vi "Stop Process VI.vi"(8 "error in (no error)":errorcluster, 9 "Blocking (T)":bool=TRUE, 10 "Process Name":string, 11 "Data in":T1={"Main VI Queue"=refnum, "Process Queue References"=[], "Message Queue"=refnum, "Visible Hardware VI"="", "Current Message"={"Source"="", "Destination"="", "Time Stamp"=timestamp(0 s since 1904-01-01), "Command"="", "Data"=variant(string "")}, "Message History"=[], "Hardware"={"Process Cache"=refnum, "Plugins"=[{"Plugin Name"="", "Controller Type"=enum."Invalid", "Control Panel Path"=path "", "Plugin Type"=enum."Optimizer"}, {"Plugin Name"="", "Controller Type"=enum."Invalid", "Control Panel Path"=path "", "Plugin Type"=enum."Optimizer"}, {"Plugin Name"="", "Controller Type"=enum."Invalid", "Control Panel Path"=path "", "Plugin Type"=enum."Optimizer"}, {"Plugin Name"="", "Controller Type"=enum."Invalid", "Control Panel Path"=path "", "Plugin Type"=enum."Optimizer"}]}, "Optimizers"={"Process Cache"=refnum, "Plugins"=[{"Plugin Name"="Deep Reaction Optimizer", "Controller Type"=enum."Invalid", "Control Panel Path"=path "", "Plugin Type"=enum."Optimizer"}, {"Plugin Name"="..\\Optimizers\\Deep Reaction Optimizer\\Control Panel\\Main.vi", "Controller Type"=enum."Invalid", "Control Panel Path"=path "", "Plugin Type"=enum."Optimizer"}, {"Plugin Name"="..\\Optimizers\\Deep Reaction Optimizer\\Source - zmq\\start_inference.bat", "Controller Type"=enum."Invalid", "Control Panel Path"=path "", "Plugin Type"=enum."Optimizer"}], "First parameters?"=FALSE, "New Parameters"={"Time Stamp"=timestamp(0 s since 1904-01-01), "Names"=[], "Values"=[]}}, "Parameter to Hardware Map"=refnum, "Analyzers"={"Process Cache"=refnum, "Plugins"=[{"Plugin Name"="ChromTech Pump Controller", "Controller Type"=enum."Invalid", "Control Panel Path"=path "", "Plugin Type"=enum."Optimizer"}, {"Plugin Name"="Pump Controller", "Controller Type"=enum."Invalid", "Control Panel Path"=path "", "Plugin Type"=enum."Optimizer"}, {"Plugin Name"="..\\Instrumentation\\ChromTech MX-Class\\Control Panel\\Main.vi", "Controller Type"=enum."Invalid", "Control Panel Path"=path "", "Plugin Type"=enum."Optimizer"}, {"Plugin Name"="", "Controller Type"=enum."Invalid", "Control Panel Path"=path "", "Plugin Type"=enum."Optimizer"}]}, "Log Directory"=path "", "Auto Pass Parameters"=FALSE, "Experiment"={"Name"="", "File Path"=path "", "File Extension"="", "File Cluster"={"Hardware List"=[], "Optimizer List"=[], "Analyzer List"=[], "Parameter to Hardware Map"=[]}}}) -> (0 "error out":errorcluster, 3 "Data out":T1={"Main VI Queue"=refnum, "Process Queue References"=[], "Message Queue"=refnum, "Visible Hardware VI"="", "Current Message"={"Source"="", "Destination"="", "Time Stamp"=timestamp(0 s since 1904-01-01), "Command"="", "Data"=variant(string "")}, "Message History"=[], "Hardware"={"Process Cache"=refnum, "Plugins"=[{"Plugin Name"="", "Controller Type"=enum."Invalid", "Control Panel Path"=path "", "Plugin Type"=enum."Optimizer"}, {"Plugin Name"="", "Controller Type"=enum."Invalid", "Control Panel Path"=path "", "Plugin Type"=enum."Optimizer"}, {"Plugin Name"="", "Controller Type"=enum."Invalid", "Control Panel Path"=path "", "Plugin Type"=enum."Optimizer"}, {"Plugin Name"="", "Controller Type"=enum."Invalid", "Control Panel Path"=path "", "Plugin Type"=enum."Optimizer"}]}, "Optimizers"={"Process Cache"=refnum, "Plugins"=[{"Plugin Name"="Deep Reaction Optimizer", "Controller Type"=enum."Invalid", "Control Panel Path"=path "", "Plugin Type"=enum."Optimizer"}, {"Plugin Name"="..\\Optimizers\\Deep Reaction Optimizer\\Control Panel\\Main.vi", "Controller Type"=enum."Invalid", "Control Panel Path"=path "", "Plugin Type"=enum."Optimizer"}, {"Plugin Name"="..\\Optimizers\\Deep Reaction Optimizer\\Source - zmq\\start_inference.bat", "Controller Type"=enum."Invalid", "Control Panel Path"=path "", "Plugin Type"=enum."Optimizer"}], "First parameters?"=FALSE, "New Parameters"={"Time Stamp"=timestamp(0 s since 1904-01-01), "Names"=[], "Values"=[]}}, "Parameter to Hardware Map"=refnum, "Analyzers"={"Process Cache"=refnum, "Plugins"=[{"Plugin Name"="ChromTech Pump Controller", "Controller Type"=enum."Invalid", "Control Panel Path"=path "", "Plugin Type"=enum."Optimizer"}, {"Plugin Name"="Pump Controller", "Controller Type"=enum."Invalid", "Control Panel Path"=path "", "Plugin Type"=enum."Optimizer"}, {"Plugin Name"="..\\Instrumentation\\ChromTech MX-Class\\Control Panel\\Main.vi", "Controller Type"=enum."Invalid", "Control Panel Path"=path "", "Plugin Type"=enum."Optimizer"}, {"Plugin Name"="", "Controller Type"=enum."Invalid", "Control Panel Path"=path "", "Plugin Type"=enum."Optimizer"}]}, "Log Directory"=path "", "Auto Pass Parameters"=FALSE, "Experiment"={"Name"="", "File Path"=path "", "File Extension"="", "File Cluster"={"Hardware List"=[], "Optimizer List"=[], "Analyzer List"=[], "Parameter to Hardware Map"=[]}}})   [LabVIEW 2020]
doc: "Stops the named process, shutting down the subpanel indicator and control panel, removing the entry from the message history cache, and deleting it form the object array. This VI triggers status update events."
uses:
  Plugin Servers/Controller Array/Controller Array.lvclass
  Type Definitions/Data.ctl
  Plugin Servers/Parameter to Hardware Map/Parameter to Hardware Map.lvclass
  <userlib>/Dynamic Reentrant/Type Defs/Message.ctl
  Plugin Manager/Plugin Details.ctl
  Plugin Servers/Controller/Controller Type.ctl
  Plugin Manager/Plugin Types.ctl
  Experiment/Experiment File/Experiment File Cluster.ctl
  Plugin Servers/Controller/Minimal Controller Cluster.ctl
  Plugin Servers/Parameter to Hardware Map/Minimal Map.ctl
  Plugin Servers/Parameter to Hardware Map/Minimal Pair Cluster.ctl
  Plugin Servers/Controller/Generic Plugin.lvclass
  <userlib>/Dynamic Reentrant/Dynamic Reentrant.lvlib
  Experiment/Experiment File/Experiment File.lvlib
  Plugin Manager/Plugin Manager.lvlib
panel:
  # "Note: Rxn Rover data control and indicator have been hidden!"
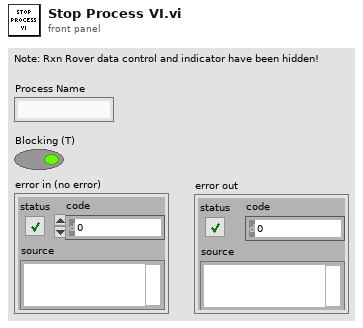
[diagram p1: front panel]
types:
  T1 = typedef "Data.ctl" = cluster{"Main VI Queue":refnum<queue>, "Process Queue References":refnum<queue>[], "Message Queue":refnum<queue>, "Visible Hardware VI":string, "Current Message":T2, "Message History":string[][], "Hardware":cluster{"Process Cache":refnum<class "Controller Array.lvclass">, "Plugins":T3[]}, "Optimizers":cluster{"Process Cache":refnum<class "Controller Array.lvclass">, "Plugins":T3[], "First parameters?":bool, "New Parameters":cluster{"Time Stamp":timestamp, "Names":string[], "Values":dbl[]}}, "Parameter to Hardware Map":refnum<class "Parameter to Hardware Map.lvclass">, "Analyzers":cluster{"Process Cache":refnum<class "Controller Array.lvclass">, "Plugins":T3[]}, "Log Directory":path, "Auto Pass Parameters":bool, "Experiment":cluster{"Name":string, "File Path":path, "File Extension":string, "File Cluster":T6}}
  T2 = typedef "Dynamic Reentrant.lvlib/Message.ctl" = cluster{"Source":string, "Destination":string, "Time Stamp":timestamp, "Command":string, "Data":variant}
  T3 = typedef "Plugin Manager.lvlib/Plugin Details.ctl" = cluster{"Plugin Name":string, "Controller Type":T4, "Control Panel Path":path, "Plugin Type":T5}
  T4 = typedef "Generic Plugin.lvclass/Controller Type.ctl" = enum16{"Invalid", "Temperature Controller", "Pump Controller", "Generic Optimizer", "LC Parser"}
  T5 = typedef "Plugin Manager.lvlib/Plugin Types.ctl" = enum16{"Invalid", "Optimizer", "Analyzer", "Hardware"}
  T6 = typedef "Experiment File.lvlib/Experiment File Cluster.ctl" = cluster{"Hardware List":T7[], "Optimizer List":T7[], "Analyzer List":T7[], "Parameter to Hardware Map":T8}
  T7 = typedef "Generic Plugin.lvclass/Minimal Controller Cluster.ctl" = cluster{"Name":string, "Controller Type":string, "Control Panel Path":string, "Resource":string}
  T8 = typedef "Parameter to Hardware Map.lvclass/Minimal Map.ctl" = T9[]
  T9 = typedef "Parameter to Hardware Map.lvclass/Minimal Pair Cluster.ctl" = cluster{"key":string, "values":T7[]}
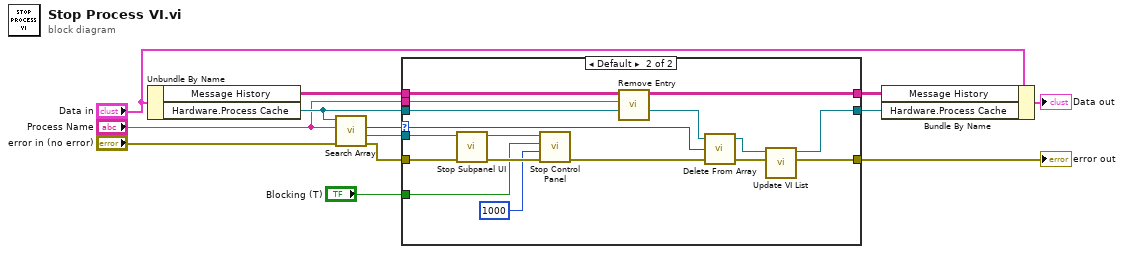
[diagram p0: block diagram]
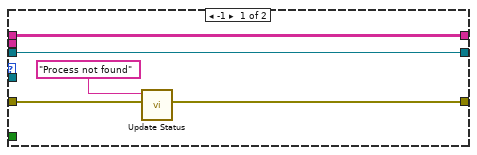
[diagram p2: hidden frame]
diagram:
  n1 = Unbundle By Name("Data in") -> ("Message History"=w7:string[][], "Hardware.Process Cache"=w8:refnum<class "Controller Array.lvclass">)
  n2 = call "Search Array.vi"("error in (no error)"="error in (no error)", "Search Value"="Process Name", "Controller Array in"=w8) -> ("error out"=w10:errorcluster, "Controller found"=w11:refnum<class "Generic Plugin.lvclass">, "Index of found"=w9:i32)  [unwired: 1 in, 1 out]
  n3 = case shown="Default" w9 {
    selector: w9 -> [_ w30]
    tunnel: [w17 w20] -> w13
    tunnel: w11 -> [_ w33]
    tunnel: w10 -> [w18 w31]
    tunnel: w8 -> [w15 w29]
    tunnel: [w15 w26] -> w3
    tunnel: w7 -> [w14 w25]
    tunnel: "Process Name" -> [_ w24]
    tunnel: [w14 w23] -> w4
    tunnel: "Blocking (T)" -> [_ w21]
    frame -1 {
      n4 = call "Update Status.vi"("error in (no error)"=w18, "Status Bar Text"="Process not found") -> ("error out"=w17:errorcluster)  [unwired: 9 in]
    }
    frame Default {
      n5 = call "Stop Subpanel UI.vi"("error in (no error)"=w31, "Controller in"=w33) -> ("error out"=w34:errorcluster, "Controller out"=w32:refnum<class "Generic Plugin.lvclass">)  [unwired: 8 in]
      n6 = call "Stop Control Panel.vi"("error in (no error)"=w34, "timeout in ms (-1)"=1000, "Blocking (T)"=w21, "controller in"=w32) -> ("error out"=w22:errorcluster)  [unwired: 6 in, 1 out]
      n7 = call "Remove Entry.vi"("Source"=w24, "Message History in"=w25) -> ("Message History out"=w23:string[][])  [unwired: 9 in]
      n8 = call "Delete From Array.vi"("error in (no error)"=w22, "index (last elem)"=w30, "Controller Array in"=w29) -> ("error out"=w27:errorcluster, "Controller Array out"=w28:refnum<class "Controller Array.lvclass">)  [unwired: 1 out]
      n9 = call "Update VI List.vi"("error in (no error)"=w27, "Controller Array in"=w28) -> ("error out"=w20:errorcluster, "Controller Array out"=w26:refnum<class "Controller Array.lvclass">)  [unwired: 8 in]
    }
  }
  "error out" <- w13
  n10 = Bundle By Name(cluster="Data in", "Message History"=w4, "Hardware.Process Cache"=w3) -> (→"Data out":T1)
